vi "Create Analog Input with Conversion Time Module.vi"(8 "error in":errorcluster, 9 "channel settings":T2[](array[typedef]), 10 "conversion time":T1, 11 "module in":refnum<class "Module.lvclass">) -> (0 "error out":errorcluster, 3 "module out":refnum<class "Module.lvclass">)   [LabVIEW 2017, in "Scan Engine Scripting.lvlib" / "Module.lvclass"]
uses:
  Module.lvclass
  Mode Classes/Controls/analog channel settings.ctl
  Mode Classes/Analog Inputs with Conversion Time Mode/Conversion Time.ctl
  Mode Classes/Analog Inputs with Conversion Time Mode/Analog Input with Conversion Time Mode.lvclass
  C:/Users/nitest/Documents/niveristand-scan-engine-ethercat-custom-device/Custom Device Source/Scripting/Modules/Mode Classes/Mode/Mode.lvclass
  C:/Users/nitest/Documents/niveristand-scan-engine-ethercat-custom-device/Custom Device Source/Scripting/Modules/Mode Classes/Analog Input Mode/Analog Input Vrms Mode/Analog Input Mode.lvclass
  Channel Classes/AI Channel/AI Channel.lvclass
  C:/Users/nitest/Documents/niveristand-scan-engine-ethercat-custom-device/Custom Device Source/Scripting/Modules/Channel Classes/Channel/Channel.lvclass
  Mode Classes/Analog Input Mode/Analog Input Vrms Mode/Analog Input Mode.lvclass
  Scan Engine Scripting.lvlib
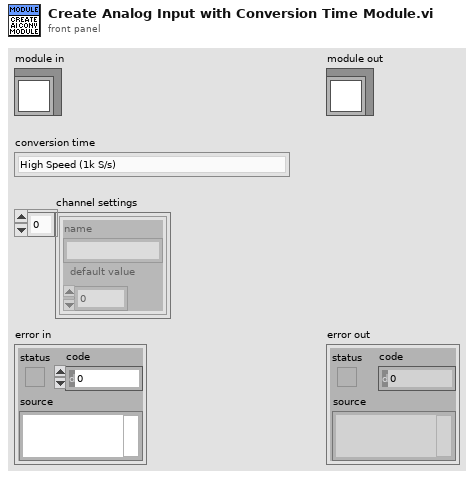
[diagram p1: front panel]
types:
  T1 = typedef "Scan Engine Scripting.lvlib/Analog Input with Conversion Time Mode.lvclass/Conversion Time.ctl" = enum16{"High Speed (1k S/s)", "Medium Speed (100 S/s)", "Medium Resolution (50/60Hz Rejection - 12 S/s)", "High Resolution (50/60Hz Rejection - 2 S/s)"}
  T2 = typedef "Scan Engine Scripting.lvlib/analog channel settings.ctl" = cluster{"name":string, "default value":dbl}
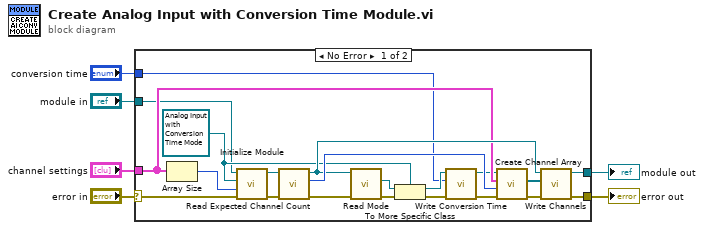
[diagram p0: block diagram]
diagram:
  n1 = case shown="No Error" "error in" {
    selector: "error in" -> [w16 w29]
    tunnel: [w15 w29] -> w5
    tunnel: [w13 w28] -> w3
    tunnel: "module in" -> [w14 w28]
    tunnel: "channel settings" -> [w17 _]
    tunnel: "conversion time" -> [w7 _]
    frame No Error {
      w18 = refnum<class "Analog Input with Conversion Time Mode.lvclass"> refnum ("Scan Engine Scripting.lvlib:Analog Input Vrms Mode.lvclass")
      n2 = Array Size(array=w17) -> (size(s)=w22:i32)
      n3 = call-dynamic "Initialize Module.vi"("error in"=w16, "channel array size"=w22, "mode"=w18, "module in"=w14) -> ("error out"=w26:errorcluster, "module out"=w27:refnum<class "Module.lvclass">)  [unwired: 6 in]
      n4 = call-dynamic "Read Expected Channel Count.vi"("error in"=w26, "module in"=w27) -> ("error out"=w20:errorcluster, "expected channel count"=w23:i32, "module out"=w21:refnum<class "Module.lvclass">)  [unwired: 7 in]
      n5 = call-dynamic "Read Mode.vi"("error in"=w20, "module in"=w21) -> ("error out"=w12:errorcluster, "mode"=w19:refnum<class "Mode.lvclass">)  [unwired: 7 in, 1 out]
      n6 = To More Specific Class(target class=w18, reference=w19, error in=w12) -> (specific class reference=w11:refnum<class "Analog Input with Conversion Time Mode.lvclass">, error out=w9:errorcluster)
      n7 = call-dynamic "Write Conversion Time.vi"("error in"=w9, "conversion time"=w7, "analog input with conversion time mode in"=w11) -> ("error out"=w8:errorcluster, "analog input with conversion time mode out"=w10:refnum<class "Analog Input with Conversion Time Mode.lvclass">)  [unwired: 7 in]
      n8 = call "Create Channel Array.vi"("error in"=w8, "expected channel count"=w23, "channel settings"=w17, "analog input mode in"=w10) -> ("error out"=w25:errorcluster, "channels"=w24:refnum<class "AI Channel.lvclass">[])  [unwired: 5 in, 1 out]
      n9 = call-dynamic "Write Channels.vi"("error in"=w25, "channels"=w24, "module in"=w21) -> ("error out"=w15:errorcluster, "module out"=w13:refnum<class "Module.lvclass">)  [unwired: 7 in]
    }
    frame Error {
    }
  }
  "error out" <- w5
  "module out" <- w3
